vi "Return Data_subVI.vi"(0 "VISA Refnum in":refnum<visa-resource-name>, 1 "Chirp Len (ms)":dbl, 2 "Amplitude (V)":dbl, 5 "Initial Freq (Hz)":dbl, 7 "Final Freq (Hz)":dbl, 9 "Interpulse Time (ms)":dbl, 11 "error in (no error)":errorcluster, 12 "Samples to Read":dbl, 13 "Iterations":dbl) -> (4 "VISA Refnum out":refnum<visa-resource-name>, 15 "error out":errorcluster)   [LabVIEW 2017]
doc: "Returns the current value of every single parameter over serial."
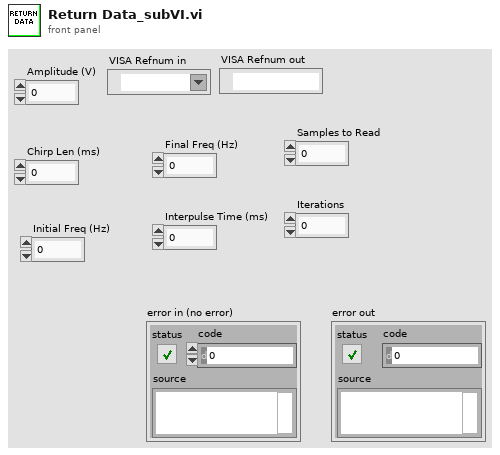
[diagram p1: front panel]
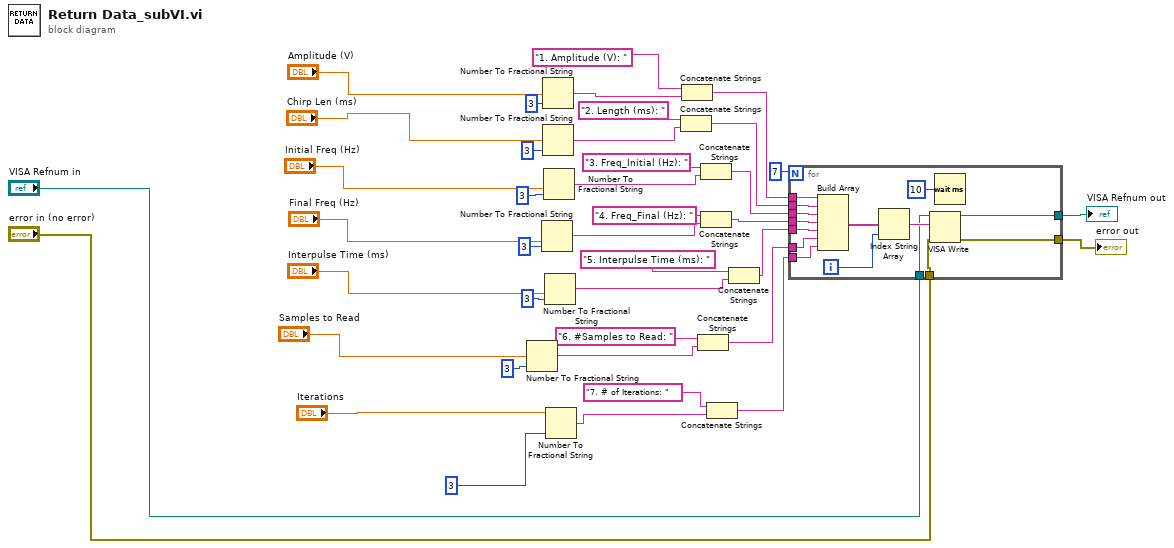
[diagram p0: block diagram]
diagram:
  n1 = Number To Fractional String(number="Samples to Read", precision (6)=i16 3) -> (F-format string=w19:string)  [unwired: 2 in]
  n2 = Number To Fractional String(number="Final Freq (Hz)", precision (6)=i16 3) -> (F-format string=w17:string)  [unwired: 2 in]
  n3 = Number To Fractional String(number="Amplitude (V)", precision (6)=i16 3) -> (F-format string=w9:string)  [unwired: 2 in]
  n4 = Number To Fractional String(number="Chirp Len (ms)", precision (6)=i16 3) -> (F-format string=w15:string)  [unwired: 2 in]
  n5 = Number To Fractional String(number="Initial Freq (Hz)", precision (6)=i16 3) -> (F-format string=w16:string)  [unwired: 2 in]
  n6 = Number To Fractional String(number="Interpulse Time (ms)", precision (6)=i16 3) -> (F-format string=w18:string)  [unwired: 2 in]
  n7 = Number To Fractional String(number="Iterations", precision (6)=i16 3) -> (F-format string=w38:string)  [unwired: 2 in]
  n8 = Concatenate Strings("2. Length (ms): " ("string"), w15) -> (w20:string)
  n9 = Concatenate Strings("1. Amplitude (V): " ("string"), w9) -> (w34:string)
  n10 = Concatenate Strings("6. #Samples to Read: " ("string"), w19) -> (w24:string)
  n11 = Concatenate Strings("3. Freq_Initial (Hz): " ("string"), w16) -> (w21:string)
  n12 = Concatenate Strings("4. Freq_Final (Hz): " ("string"), w17) -> (w22:string)
  n13 = Concatenate Strings("7. # of Iterations: " ("string"), w38) -> (w40:string)
  n14 = Concatenate Strings("5. Interpulse Time (ms): " ("string"), w18) -> (w23:string)
  n15 = for {
    N: 7 -> [_]
    tunnel: w20 -> [w55]
    tunnel: w21 -> [w54]
    tunnel: w22 -> [w53]
    tunnel: w23 -> [w52]
    tunnel: w24 -> [w42]
    tunnel: "VISA Refnum in" -> [w48]
    tunnel: "error in (no error)" -> [w47]
    tunnel: [w46] -> w25
    tunnel: [w45] -> w26
    tunnel: w34 -> [w44]
    tunnel: w40 -> [w41]
    i -> [w50]
    n16 = Build Array(w44, w55, w54, w53, w52, w42, w41) -> (w51:string[])
    n17 = Index String Array(1:w50, 2:w51) -> (0:w49:string)  [unwired: 1 in]
    n18 = VISA Write(VISA resource name=w48, write buffer=w49, error in (no error)=w47) -> (VISA resource name out=w46:refnum<visa-resource-name>, error out=w45:errorcluster)  [unwired: 1 out]
    n19 = Wait (ms)(milliseconds to wait=u32 10) -> ()  [unwired: 1 out]
  }
  "error out" <- w26
  "VISA Refnum out" <- w25
